vi "Test Comm Multi.vi"() -> ()   [LabVIEW 2021]
uses:
  CIFChannels/Typedef/Direction.ctl
  ChannelCommon/typedef/FIFO Config.ctl
  ChannelCommon/typedef/TimeStamps.ctl
  CIF_NIChn_CAN.lvclass
  D:/dev/Packages/Channel_Manager/src/CIF_NIChn/FIFO_U8/CIF_NIChn_Fifo_U8.lvclass
  D:/dev/Packages/Channel_Manager/src/CIF_NIChn/FIFO_U8_Multi/CIF_Fifo_U8_Multi.lvclass
  D:/dev/Packages/Channel_Manager/src/CIFChannels/CIFChannels.lvclass
  ChannelCommon/typedef/New FIFO Instance Configuration.ctl
  CIFChannels/CIFChannels.lvclass/CIFChannels.ctl
  <vilib>/CIF Foundation/CIF Utilities/DataTypes/Flatten U64.vi
  CIFChannels/CIFChannels.lvclass
  FIFO_U8_Multi/CIF_Fifo_U8_Multi.lvclass
  FIFO_U8/CIF_NIChn_Fifo_U8.lvclass
  ChannelCommon/ChannelCommon.lvlib
  D:/dev/Packages/Channel_Manager/src/CIF_NIChn/NIChn/CIF_NIChn.lvclass
  D:/dev/Packages/Channel_Manager/src/CIF_NIChn/FIFO_CAN/CIF_NIChn_CAN.lvclass
panel:
  out "status":string
  out "pass":bool
  out "error out":errorcluster
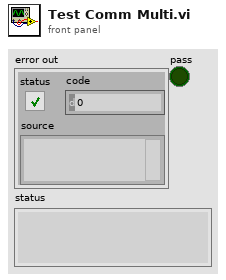
[diagram p1: front panel]
types:
  T1 = typedef "CIFChannels.lvclass/Direction.ctl" = enum16{"Publisher", "Subscriber"}
  T2 = typedef "ChannelCommon.lvlib/New FIFO Instance Configuration.ctl" = cluster{"Primary":bool, "Backpressure":bool, "Message/FIFO Override":u32}
  T3 = typedef "ChannelCommon.lvlib/TimeStamps.ctl" = cluster{"ClockID":u8, "T0":i64, "T_Out":i64}
  T4 = typedef "ChannelCommon.lvlib/FIFO Config.ctl" = cluster{"Max Bytes/Msg":u64, "Max Msg/FIFO":u64, "Flags":u64}
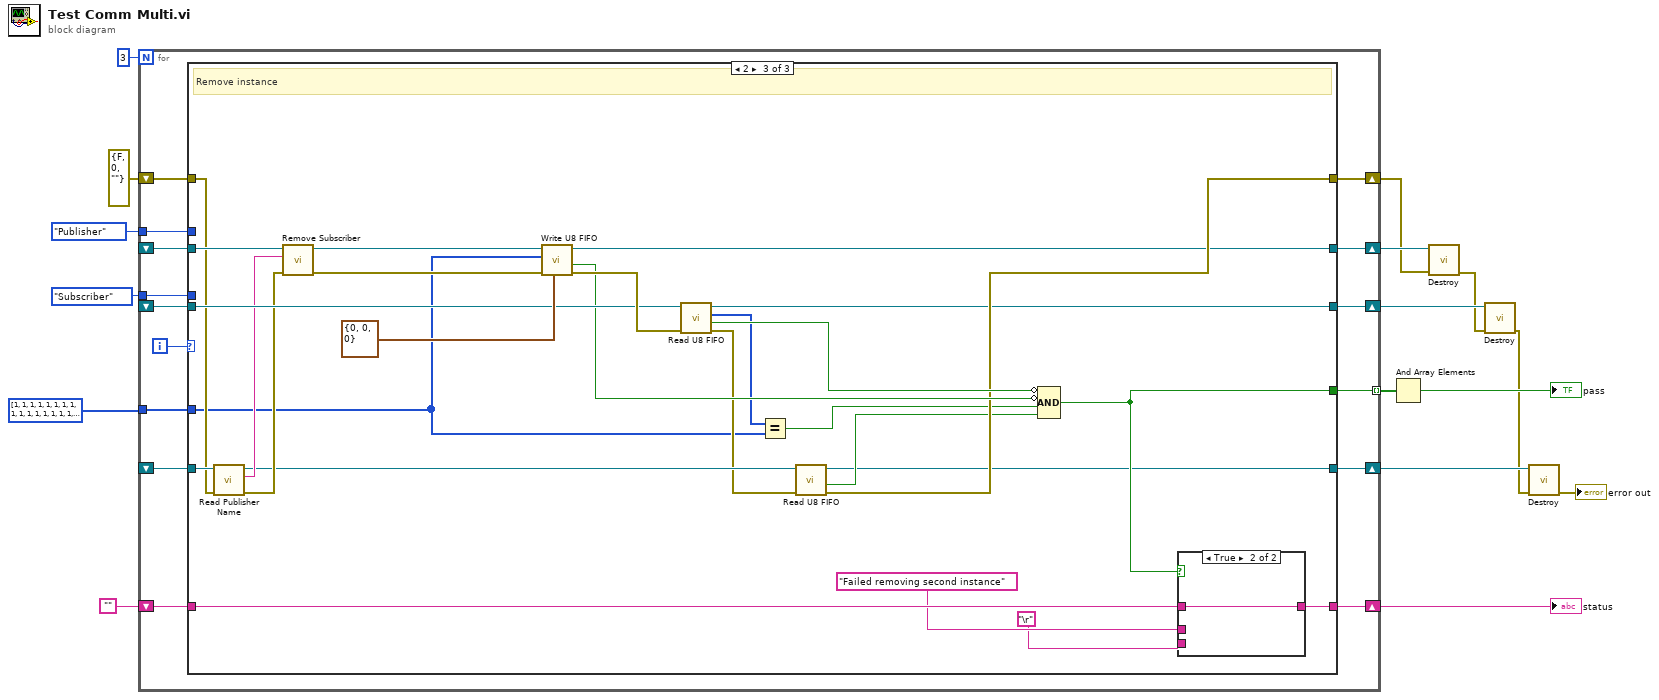
[diagram p0: block diagram]
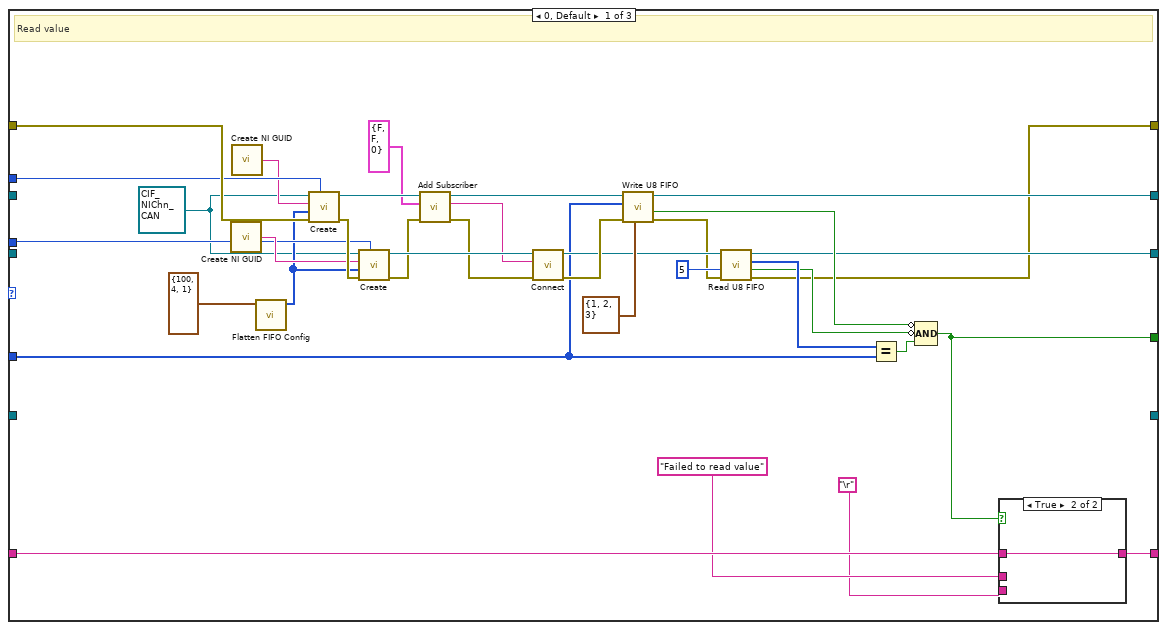
[diagram p2: hidden frame]
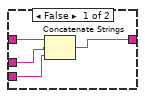
[diagram p3: hidden frame]
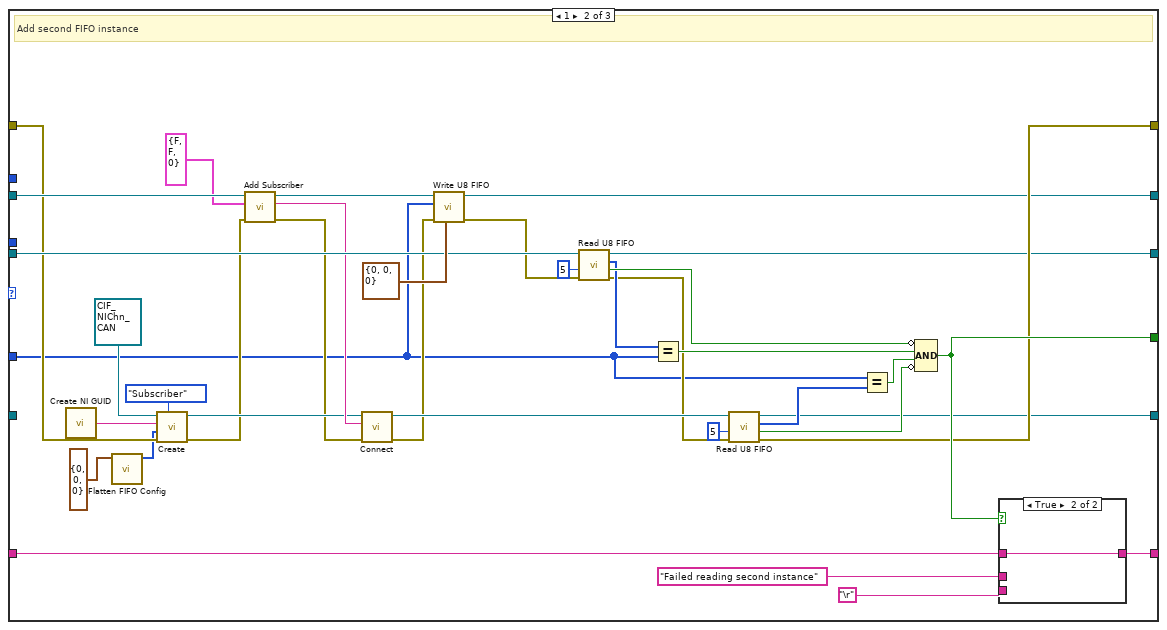
[diagram p4: hidden frame]
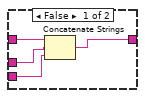
[diagram p5: hidden frame]
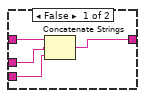
[diagram p6: hidden frame]
diagram:
  n1 = for {
    N: 3 -> [_]
    tunnel: [w31] -> w16 mode=indexing
    shift-right: [w23] -> w6
    shift-left: errorcluster {"status"=FALSE, "code"=0, "source"=""} ("error out") -> [w30]
    shift-right: [w27] -> w12
    shift-left: "" -> [w28]
    tunnel: Direction."Subscriber" ("Direction") -> [w26]
    tunnel: Direction."Publisher" ("Direction") -> [w25]
    shift-right: [w17] -> w8
    shift-left: _ -> [w21]
    shift-right: [w24] -> w7
    shift-left: _ -> [w22]
    tunnel: u8[] [1, 1, 1, 1, 1, 1, 1, 1, 1, 1, 1, 1, 1, 1, 1, 1, 1, 1, 1, 1, 1, 1, 1, 1, 1, 1, 1, 1, 1, 1, 1, 1, 1, 1, 1, 1, 1, 1, 1, 1, 1, 1, 1, 1, 1, 1, 1, 1, 1, 1, 1, 1, 1, 1, 1, 1, 1, 1, 1, 1, 1, 1, 1, 1] ("Data in") -> [w20]
    shift-right: [w18] -> w4
    shift-left: _ -> [w19]
    i -> [w29]
    n2 = case shown="2" w29 {
      tunnel: [w60 w103 w133] -> w31
      tunnel: w30 -> [w58 w87 w127]
      tunnel: [w41 w78 w120] -> w23
      tunnel: w28 -> [w65 w107 w139]
      tunnel: [w64 w106 w138] -> w27
      tunnel: w26 -> [w56 _ _]
      tunnel: w25 -> [w55 _ _]
      tunnel: [w43 w71 w114] -> w17
      tunnel: [w48 w72 w115] -> w24
      tunnel: w22 -> [_ w95 w130]
      tunnel: w21 -> [_ w96 w131]
      tunnel: w20 -> [w33 w77 w116]
      tunnel: w19 -> [_ _ w128]
      tunnel: [_ w73 w113] -> w18
      frame 0, Default {
        w40 = refnum<class "CIF_NIChn_CAN.lvclass"> refnum ("CIF_DAQ_DVR_Multi.lvclass")
        # "Read value"
        n3 = call <vilib>:"Create NI GUID.vi"() -> ("NI GUID"=w57:string)
        n4 = call <vilib>:"Create NI GUID.vi"() -> ("NI GUID"=w53:string)
        n5 = call "Flatten FIFO Config.vi"("FIFO Config in"=T4 {"Max Bytes/Msg"=100, "Max Msg/FIFO"=4, "Flags"=1}) -> ("Flattened FIFO Config"=w51:u8[])  [unwired: 10 in]
        n6 = call-dynamic "Create.vi"("Direction"=w55, "error in (no error)"=w58, "Custom Config Data"=w51, "Name"=w53, "CIF_Fifo_U8 in"=w40) -> ("error out"=w59:errorcluster, "CIF_Fifo_U8 out"=w39:refnum<class "CIF_NIChn_CAN.lvclass">)  [unwired: 5 in]
        n7 = call-dynamic "Create.vi"("Direction"=w56, "error in (no error)"=w59, "Custom Config Data"=w51, "Name"=w57, "CIF_Fifo_U8 in"=w40) -> ("error out"=w36:errorcluster, "CIF_Fifo_U8 out"=w52:refnum<class "CIF_NIChn_CAN.lvclass">)  [unwired: 5 in]
        n8 = call-dynamic "Add Subscriber.vi"("error in (no error)"=w36, "New FIFO Instance Config"=T2 {"Primary"=FALSE, "Backpressure"=FALSE, "Message/FIFO Override"=0}, "CIF_Fifo_U8 in"=w39) -> ("error out"=w35:errorcluster, "New Publisher"=w37:string, "CIF_Fifo_U8 out"=w38:refnum<class "CIF_NIChn_CAN.lvclass">)  [unwired: 6 in]
        n9 = call-dynamic "Connect.vi"("error in (no error)"=w35, "Connection Name"=w37, "CIFTag in"=w52) -> ("error out"=w50:errorcluster, "CIFTag out"=w46:refnum<class "CIF_NIChn_CAN.lvclass">)  [unwired: 7 in]
        n10 = call-dynamic "Write U8 FIFO.vi"("FIFO Timestamps"=T3 {"ClockID"=1, "T0"=2, "T_Out"=3}, "error in (no error)"=w50, "Data in"=w33, "CIF_Fifo_U8 in"=w38) -> ("error out"=w32:errorcluster, "timed out?"=w47:bool, "CIF_Fifo_U8 out"=w48:refnum<class "CIF_NIChn_CAN.lvclass">)  [unwired: 4 in, 1 out]
        n11 = call-dynamic "Read U8 FIFO.vi"("error in (no error)"=w32, "Timeout (ms)"=5, "CIFFIFO in"=w46) -> ("error out"=w41:errorcluster, "timed out?"=w42:bool, "Data out"=w44:u8[], "CIFFIFO out"=w43:refnum<class "CIF_NIChn_CAN.lvclass">)  [unwired: 4 in, 1 out]
        n12 = Equal?(x=w44, y=w33) -> (x = y?=w61:bool)
        n13 = Compound Arithmetic op=AND(invert w47, invert w42, w61) -> (w60:bool)
        n14 = case shown="True" w60 {
          tunnel: w65 -> [w69 w70]
          tunnel: [w66 w70] -> w64
          tunnel: "Failed to read value" -> [w68 _]
          tunnel: "\r" -> [w67 _]
          frame False {
            n15 = Concatenate Strings(w69, w68, w67) -> (w66:string)
          }
          frame True {
          }
        }
      }
      frame 1 {
        # "Add second FIFO instance"
        n16 = call <vilib>:"Create NI GUID.vi"() -> ("NI GUID"=w92:string)
        n17 = call "Flatten FIFO Config.vi"("FIFO Config in"=T4 {"Max Bytes/Msg"=0, "Max Msg/FIFO"=0, "Flags"=0}) -> ("Flattened FIFO Config"=w86:u8[])  [unwired: 10 in]
        n18 = call-dynamic "Create.vi"("Direction"=Direction."Subscriber", "error in (no error)"=w87, "Custom Config Data"=w86, "Name"=w92, "CIF_Fifo_U8 in"=refnum<class "CIF_NIChn_CAN.lvclass"> refnum ("CIF_DAQ_DVR_Multi.lvclass")) -> ("error out"=w88:errorcluster, "CIF_Fifo_U8 out"=w90:refnum<class "CIF_NIChn_CAN.lvclass">)  [unwired: 5 in]
        n19 = call-dynamic "Add Subscriber.vi"("error in (no error)"=w88, "New FIFO Instance Config"=T2 {"Primary"=FALSE, "Backpressure"=FALSE, "Message/FIFO Override"=0}, "CIF_Fifo_U8 in"=w95) -> ("error out"=w89:errorcluster, "New Publisher"=w91:string, "CIF_Fifo_U8 out"=w94:refnum<class "CIF_Fifo_U8_Multi.lvclass">)  [unwired: 6 in]
        n20 = call-dynamic "Connect.vi"("error in (no error)"=w89, "Connection Name"=w91, "CIFTag in"=w90) -> ("error out"=w81:errorcluster, "CIFTag out"=w82:refnum<class "CIF_NIChn_CAN.lvclass">)  [unwired: 7 in]
        n21 = call-dynamic "Write U8 FIFO.vi"("FIFO Timestamps"=T3 {"ClockID"=0, "T0"=0, "T_Out"=0}, "error in (no error)"=w81, "Data in"=w77, "CIF_Fifo_U8 in"=w94) -> ("error out"=w76:errorcluster, "CIF_Fifo_U8 out"=w72:refnum<class "CIF_Fifo_U8_Multi.lvclass">)  [unwired: 4 in, 2 out]
        n22 = call-dynamic "Read U8 FIFO.vi"("error in (no error)"=w76, "Timeout (ms)"=5, "CIFFIFO in"=w96) -> ("error out"=w79:errorcluster, "timed out?"=w99:bool, "Data out"=w98:u8[], "CIFFIFO out"=w71:refnum<class "CIF_NIChn_Fifo_U8.lvclass">)  [unwired: 4 in, 1 out]
        n23 = Equal?(x=w98, y=w77) -> (x = y?=w101:bool)
        n24 = call-dynamic "Read U8 FIFO.vi"("error in (no error)"=w79, "Timeout (ms)"=5, "CIFFIFO in"=w82) -> ("error out"=w78:errorcluster, "timed out?"=w74:bool, "Data out"=w80:u8[], "CIFFIFO out"=w73:refnum<class "CIF_NIChn_CAN.lvclass">)  [unwired: 4 in, 1 out]
        n25 = Equal?(x=w77, y=w80) -> (x = y?=w102:bool)
        n26 = Compound Arithmetic op=AND(invert w99, w101, w102, invert w74) -> (w103:bool)
        n27 = case shown="True" w103 {
          tunnel: w107 -> [w111 w112]
          tunnel: [w108 w112] -> w106
          tunnel: "Failed reading second instance" -> [w110 _]
          tunnel: "\r" -> [w109 _]
          frame False {
            n28 = Concatenate Strings(w111, w110, w109) -> (w108:string)
          }
          frame True {
          }
        }
      }
      frame 2 {
        # "Remove instance"
        n29 = call "Read Publisher Name.vi"("error in (no error)"=w127, "CIFChannels in"=w128) -> ("error out"=w124:errorcluster, "Publisher Name"=w126:string, "CIFChannels out"=w122:refnum<class "CIF_NIChn_CAN.lvclass">)  [unwired: 7 in]
        n30 = call-dynamic "Remove Subscriber.vi"("error in (no error)"=w124, "Publisher to Remove"=w126, "CIF_Fifo_U8 in"=w130) -> ("error out"=w125:errorcluster, "CIF_Fifo_U8 out"=w129:refnum<class "CIF_Fifo_U8_Multi.lvclass">)  [unwired: 7 in]
        n31 = call-dynamic "Write U8 FIFO.vi"("FIFO Timestamps"=T3 {"ClockID"=0, "T0"=0, "T_Out"=0}, "error in (no error)"=w125, "Data in"=w116, "CIF_Fifo_U8 in"=w129) -> ("error out"=w135:errorcluster, "timed out?"=w123:bool, "CIF_Fifo_U8 out"=w115:refnum<class "CIF_Fifo_U8_Multi.lvclass">)  [unwired: 4 in, 1 out]
        n32 = call-dynamic "Read U8 FIFO.vi"("error in (no error)"=w135, "CIFFIFO in"=w131) -> ("error out"=w121:errorcluster, "timed out?"=w134:bool, "Data out"=w119:u8[], "CIFFIFO out"=w114:refnum<class "CIF_NIChn_Fifo_U8.lvclass">)  [unwired: 5 in, 1 out]
        n33 = Equal?(x=w119, y=w116) -> (x = y?=w118:bool)
        n34 = call-dynamic "Read U8 FIFO.vi"("error in (no error)"=w121, "CIFFIFO in"=w122) -> ("error out"=w120:errorcluster, "timed out?"=w117:bool, "CIFFIFO out"=w113:refnum<class "CIF_NIChn_CAN.lvclass">)  [unwired: 5 in, 2 out]
        n35 = Compound Arithmetic op=AND(invert w134, invert w123, w118, w117) -> (w133:bool)
        n36 = case shown="True" w133 {
          tunnel: w139 -> [w143 w144]
          tunnel: [w140 w144] -> w138
          tunnel: "Failed removing second instance" -> [w142 _]
          tunnel: "\r" -> [w141 _]
          frame False {
            n37 = Concatenate Strings(w143, w142, w141) -> (w140:string)
          }
          frame True {
          }
        }
      }
    }
  }
  "status" <- w12
  n38 = And Array Elements(Boolean array=w16) -> (logical AND=→"pass":bool)
  n39 = call-dynamic "Destroy.vi"("error in (no error)"=w6, "CIF_Fifo_U8 in"=w7) -> ("error out"=w5:errorcluster)  [unwired: 8 in, 1 out]
  n40 = call-dynamic "Destroy.vi"("error in (no error)"=w5, "CIFFIFO in"=w8) -> ("error out"=w3:errorcluster)  [unwired: 8 in, 1 out]
  n41 = call-dynamic "Destroy.vi"("error in (no error)"=w3, "CIF_Fifo_U8 in"=w4) -> ("error out"=→"error out":errorcluster)  [unwired: 8 in, 1 out]
